vi "database element to configuration object.vi"(8 "error in":errorcluster, 11 "database":T1) -> (0 "error out":errorcluster, 3 "configuration in":refnum<class "TBM configuration.lvclass">)   [LabVIEW 2013, in "PLConfigurationSerializer.lvlib"]
uses:
  PLConfigurationSerializer.lvlib
  <vilib>/NI/Tag Bus Module Framework/root configuration/TBM configuration.lvclass
  configuration database.ctl
  plugin discovery singleton/class discovery singleton methods.ctl
  plugin discovery singleton/class discovery singleton.lvlib
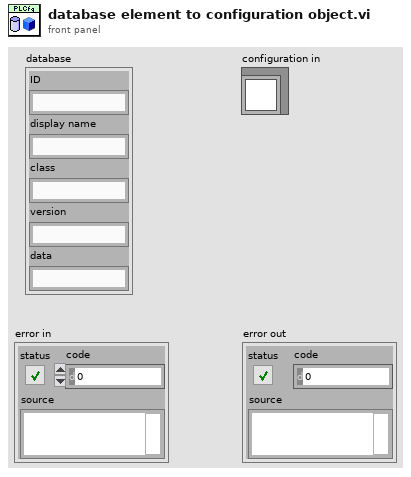
[diagram p1: front panel]
types:
  T1 = typedef "PLConfigurationSerializer.lvlib/configuration database.ctl" = cluster{"ID":string, "display name":string, "class":string, "version":string, "data":string}
  T2 = typedef "class discovery singleton.lvlib/class discovery singleton methods.ctl" = enum16{"add search paths", "load class by name", "list available classes", "get class path"}
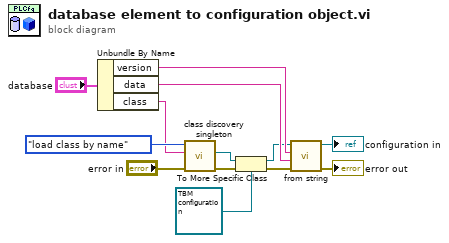
[diagram p0: block diagram]
diagram:
  n1 = Unbundle By Name("database") -> ("version"=w12:string, "data"=w11:string, "class"=w8:string)
  n2 = call "class discovery singleton.vi"("error in"="error in", "Class Name"=w8, "method"=class_discovery_singleton_methods."load class by name") -> ("error out"=w10:errorcluster, "LabVIEW Object"=w6:refnum<class>)  [unwired: 5 in, 2 out]
  n3 = To More Specific Class(target class=refnum<class "TBM configuration.lvclass"> refnum ("configuration in"), reference=w6, error in=w10) -> (specific class reference=w4:refnum<class "TBM configuration.lvclass">, error out=w7:errorcluster)
  n4 = call-dynamic "from string.vi"("error in"=w7, "data"=w11, "version"=w12, "configuration in"=w4) -> ("error out"=→"error out":errorcluster, "configuration out"=→"configuration in":refnum<class "TBM configuration.lvclass">)  [unwired: 6 in]
